vi "Convert Non-visible Char to Visible Char.vi"(7 "append ASCII column?":bool=TRUE, 10 "bytes per row":i32=8, 11 "data":u8[](array[numeric])=[255, 255, 255, 255, 255, 255, 255, 255, 255, 255, 255, 255, 255, 255, 255, 255, 255, 255, 255, 255, 255, 255, 255, 255, 255, 255, 255, 255, 255, 255, 255, 255, 255, 255, 255, 255, 255, 255, 255, 255, 255, 255, 255, 255, 255, 255, 255, 255, 255, 255, 255, 255, 255, 255, 255, 255, 255, 255, 255, 255, 255, 255, 255, 255, 255, 255, 255, 255, 255, 255, 255, 255, 255, 255, 255, 255, 255, 255, 255, 255, 255, 255, 255, 255, 255, 255, 255, 255, 255, 255, 255, 255, 255, 255, 255, 255, 255, 255, 255, 170] format="%.0x") -> (1 "last row":u8[](array[numeric]) format="%.0x", 2 "output array":u8[][](array[numeric]) format="%.0x", 3 "data table":string[][](table))   [LabVIEW 2020, in "FrameEditor.lvlib"]
uses:
  FrameEditor.lvlib
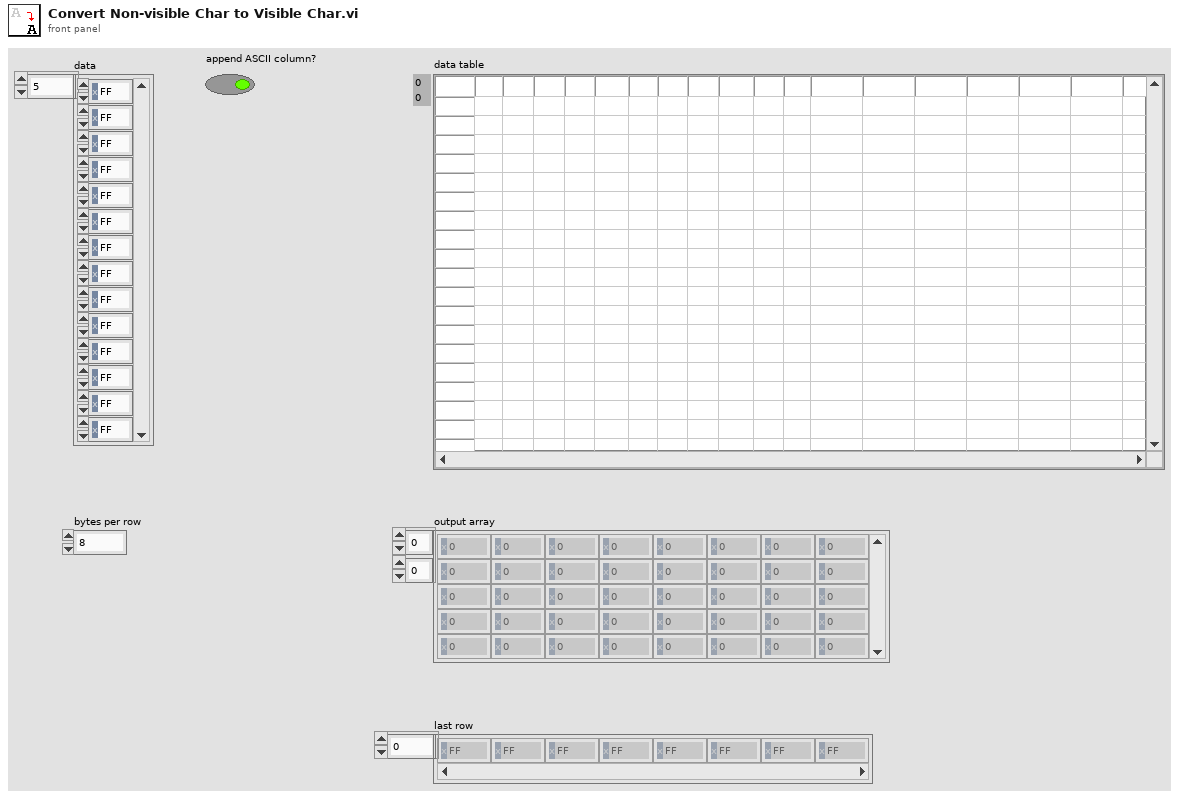
[diagram p1: front panel]
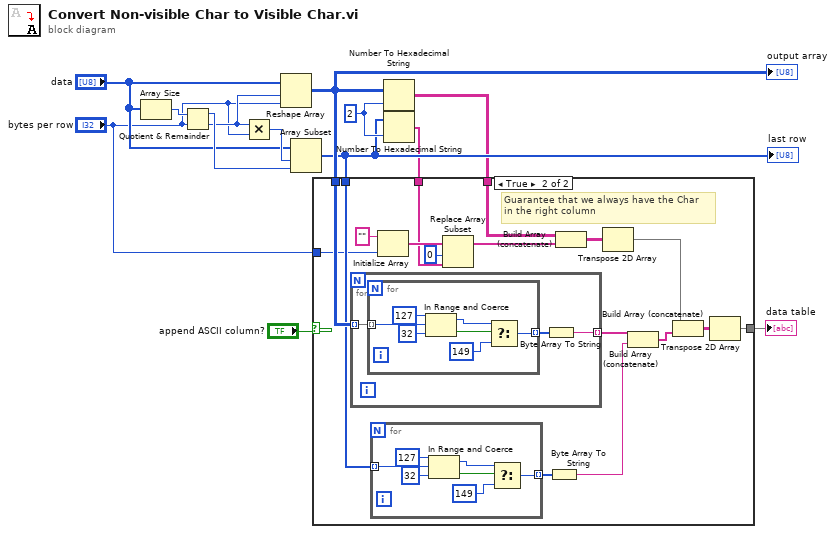
[diagram p0: block diagram]
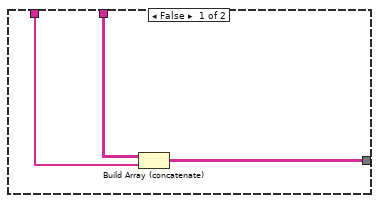
[diagram p2: hidden frame]
diagram:
  w5 = i16 2 ("width (-)")
  n1 = Array Size(array="data") -> (size(s)=w13:i32)
  n2 = Quotient & Remainder(x=w13, y="bytes per row") -> (x-y*floor(x/y)=w12:i32, floor(x/y)=w9:i32)
  n3 = Multiply(x=w9, y="bytes per row") -> (x*y=w11:i32)
  n4 = Reshape Array("data", w9, "bytes per row") -> (w8:u8[][])
  "output array" <- w8
  n5 = Array Subset(array="data", index=w11, length=w12) -> (w4:u8[])
  "last row" <- w4
  n6 = Number To Hexadecimal String(1:w5, 2:w8) -> (0:w1:string[][])
  n7 = Number To Hexadecimal String(1:w5, 2:w4) -> (0:w2:string[])
  n8 = case shown="True" "append ASCII column?" {
    tunnel: w8 -> [_ w33]
    tunnel: [w14 w31] -> w7
    tunnel: w4 -> [_ w29]
    tunnel: "bytes per row" -> [_ w22]
    tunnel: w2 -> [w16 w21]
    tunnel: w1 -> [w15 w19]
    frame False {
      n9 = Build Array (concatenate)(w15, w16) -> (w14:string[][])
    }
    frame True {
      # "Guarantee that we always have the Char\nin the right column"
      n10 = for {
        tunnel: w33 -> [w43] mode=indexing
        tunnel: [w41] -> w28 mode=indexing
        n11 = for {
          tunnel: w43 -> [w50] mode=indexing
          tunnel: [w44] -> w42 mode=indexing
          n12 = In Range and Coerce(upper limit=u8 127, x=w50, lower limit=u8 32) -> (coerced(x)=w48:u8, In Range?=w49:bool)
          n13 = Select(t=w48, s=w49, f=u8 149) -> (s? t:f=w44:u8)
        }
        n14 = Byte Array To String(unsigned byte array=w42) -> (string=w41:string)
      }
      n15 = for {
        tunnel: w29 -> [w40] mode=indexing
        tunnel: [w34] -> w30 mode=indexing
        n16 = In Range and Coerce(upper limit=u8 127, x=w40, lower limit=u8 32) -> (coerced(x)=w38:u8, In Range?=w39:bool)
        n17 = Select(t=w38, s=w39, f=u8 149) -> (s? t:f=w34:u8)
      }
      n18 = Initialize Array("" ("string"), w22) -> (w24:string[])
      n19 = Replace Array Subset(array=w24, new element=w21, index=0) -> (w17:string[])
      n20 = Byte Array To String(unsigned byte array=w30) -> (string=w27:string)
      n21 = Build Array (concatenate)(w19, w17) -> (w18:string[][])
      n22 = Transpose 2D Array(2D array=w18) -> (transposed array=w25:string[][])
      n23 = Build Array (concatenate)(w28, w27) -> (w26:string[])
      n24 = Build Array (concatenate)(w25, w26) -> (w32:string[][])
      n25 = Transpose 2D Array(2D array=w32) -> (transposed array=w31:string[][])
    }
  }
  "data table" <- w7
